vi "Puff_Release_Decay.vi"() -> (5 "Plug in titles":string[](array[string]), 7 "Plug in values":string[](array[string]))   [LabVIEW 2012]
uses:
  Globals/Meas_global.vi
  <vilib>/Analysis/baseanly.llb/Mean (DBL).vi
  <vilib>/Analysis/NI_AALBase.lvlib
  <vilib>/Analysis/NI_AALPro.lvlib
panel:
  out "Mean Concentration":dbl
  out "element":string
  out "index of element":i32
  out "Array":path[](array[path])
  out "tau":dbl(graph)
  out "tau (s)":dbl[](array[numeric])=[nan]
  in  "Median filter passes":i32=1
  in  "Median filter extent":i32=20
  in  "Normalised multiplot":bool
  in  "Cut at start":i32=200
  in  "Keep after cut":i32=2800
  in  "min threshold":dbl=4.0
  in  "Reset":bool
  out "Current Block No":i32=51
  out "Multiplot":T1(graph)
  out "XY Graph":cluster{"Time (ms)":dbl[], dbl[]}(graph)
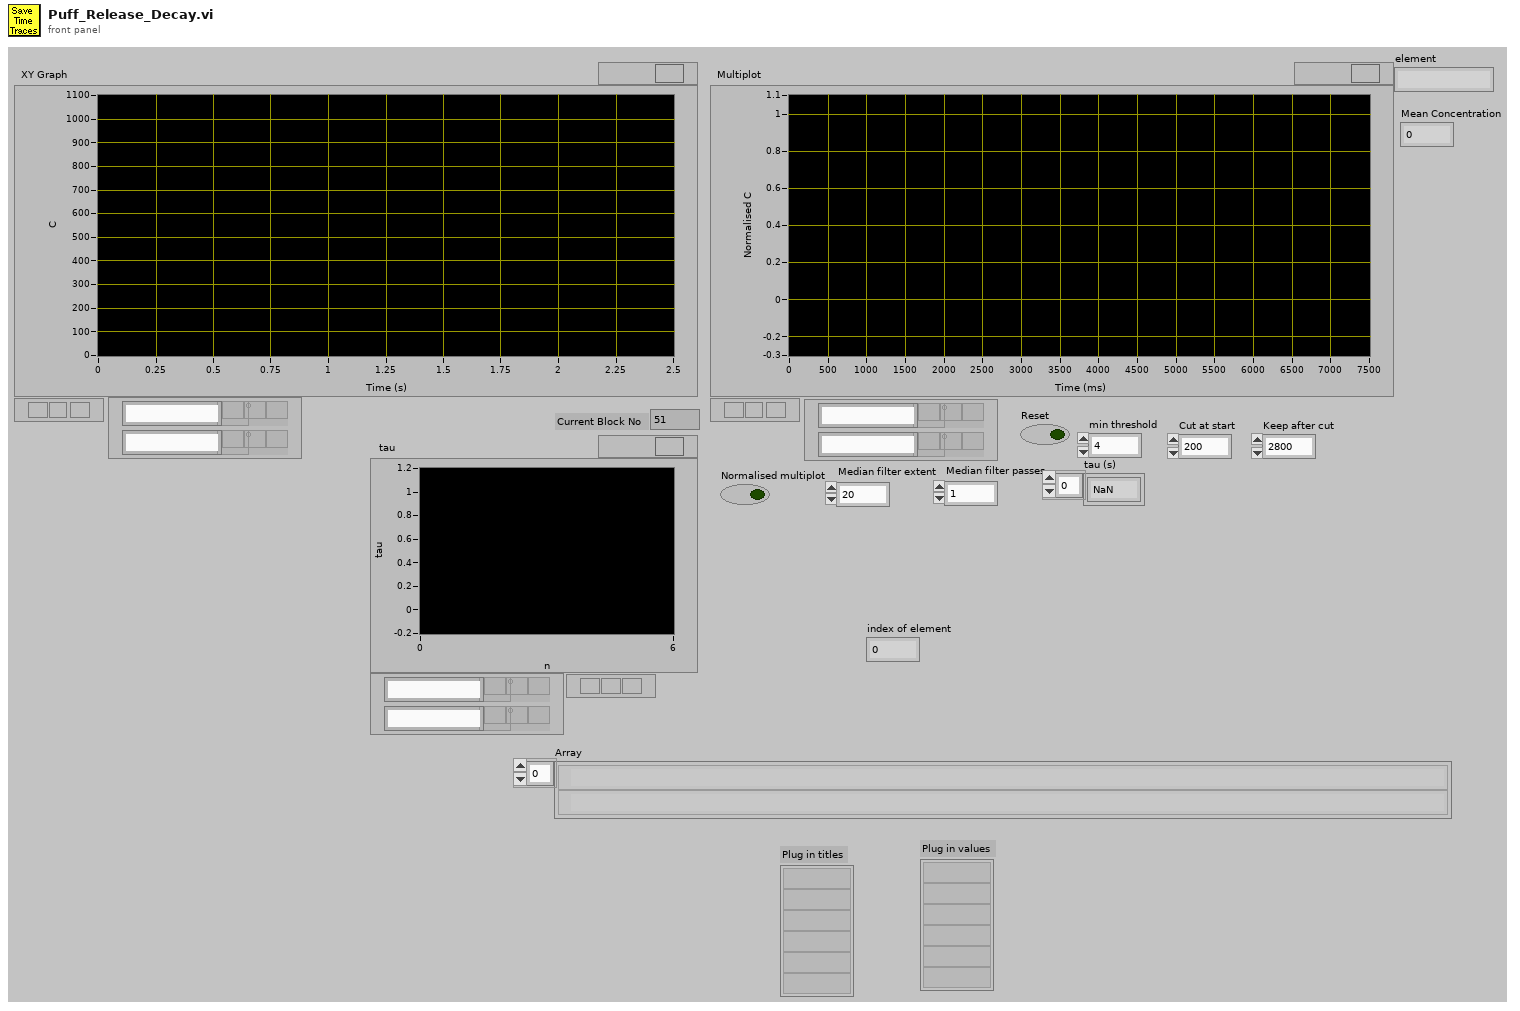
[diagram p1: front panel]
types:
  T1 = cluster{"Time (ms)":dbl[], "Y[i]=X[i]/Max|X|":dbl[]}[]
  T2 = typedef "Analysis_info_cluster.ctl" = cluster{"Colour":u32, "Inst type":T3, "Inst name":string, "Symbol":string, "Code name":string, "Extra Info":string, "Inst Array":T4, "Extra Titles":string[], "Extra Values":string[], "U":dbl, "u^2":dbl, "u^3":dbl, "u^4":dbl, "Skew_u":dbl, "Kurt_u":dbl, "Sd Error in Mean":dbl, "% u'/U":dbl, "X":dbl, "Y":dbl, "Z":dbl, "Timescale integral to 25%":dbl, "Sd Error in Variance":dbl, "Calib File":path, "Calib Constants":dbl[], "Output Position":bool, "Full Stats":bool, "Av Sampling Rate":dbl, "Av No of Samples":dbl, "Total Meas Time (s)":dbl, "ADAM Ch Name":string}
  T3 = typedef "Inst_type.ctl" = enum16{"Propeller anemometer", "Raw voltage", "Pressure Transducer", "Pitot-static tube", "Preston tube", "Hot wire", "Cross wire 1", "Cross wire 2", "Generic Linear", "Generic Polynomial", "Generic BackPoly", "Fast FID", "Thermocouple", "Cold wire", "Pulsed Wire", "LDA Vel", "LDA Tran time", "LDA Arr time"}
  T4 = typedef "Instrument_Array.ctl" = enum16{"PWA", "LDA", "Analogue"}
  T5 = typedef "Time_Trace_Cluster.ctl" = cluster{"Weighting":dbl[], "Time (s)":dbl[], "Voltage":dbl[], "Eng Values":dbl[]}
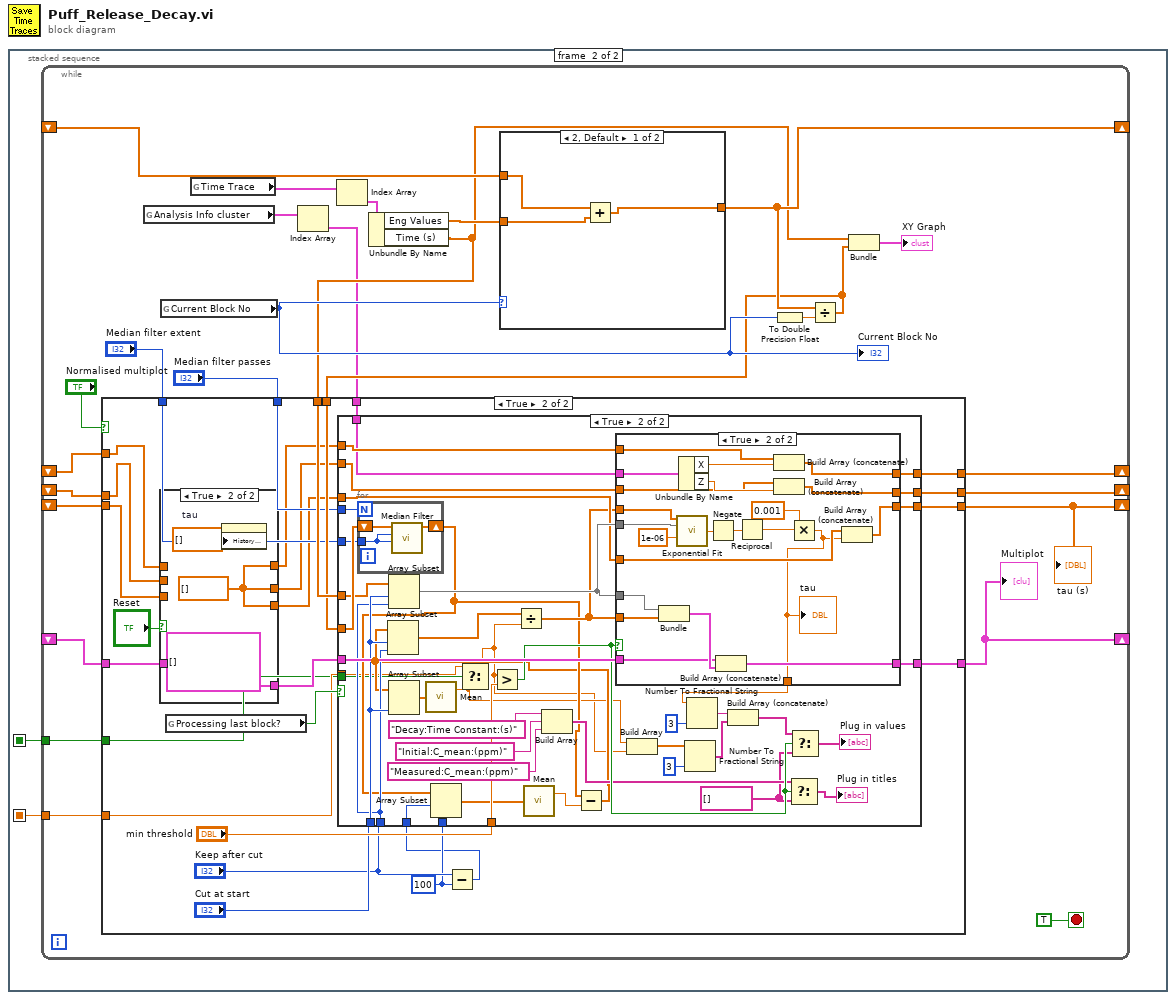
[diagram p0: block diagram]
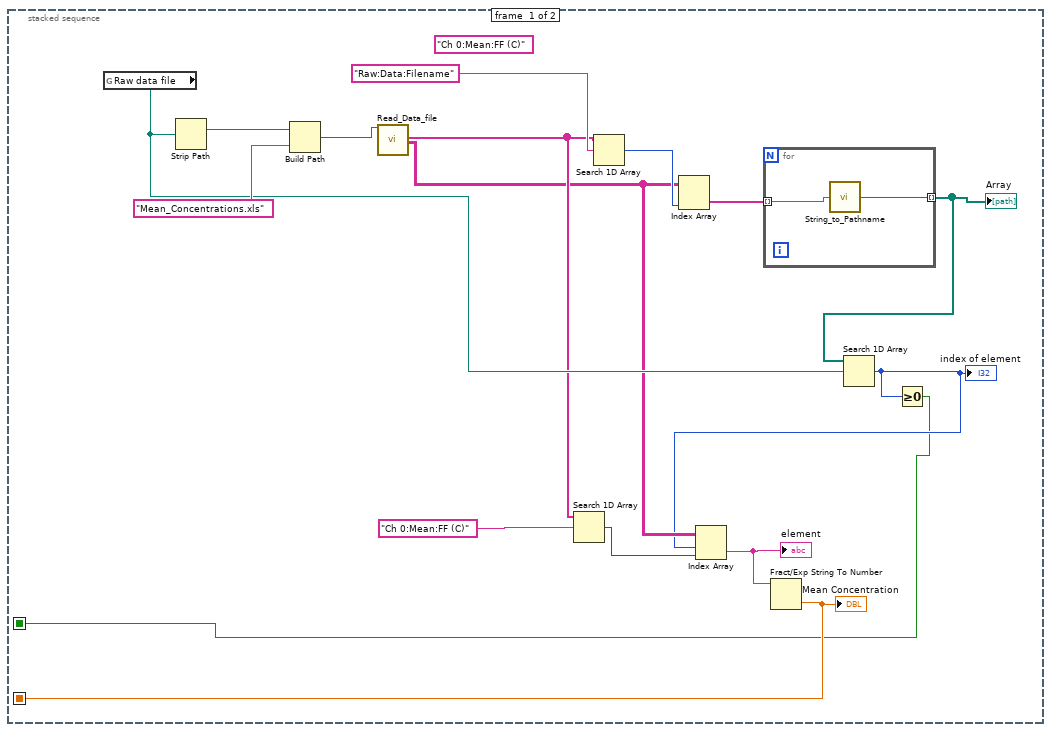
[diagram p2: hidden frame]
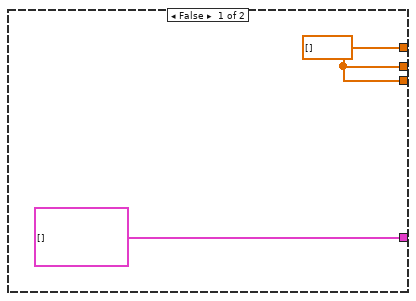
[diagram p3: hidden frame]
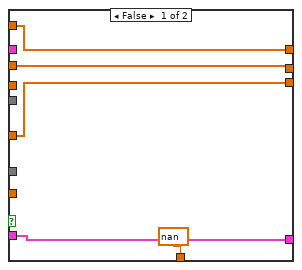
[diagram p6: hidden frame]
diagram:
  n1 = stacked-sequence {
    seq-local: [w3 _] -> [_ w20]
    seq-local: [w1 _] -> [_ w19]
    frame #0 {
      (unwired) "Ch 0:Mean:FF (C)"
      n2 = global read "Meas_global.vi" "Raw data file"() -> (w9:path)
      n3 = Strip Path(path=w9) -> (stripped path=w16:path)  [unwired: 1 out]
      n4 = Build Path(base path=w16, name or relative path="Mean_Concentrations.xls") -> (appended path=w14:path)
      n5 = call "Read_Data_file.vi"("Results file"=w14) -> ("Ch names Out"=w8:string[], "Channel Values Out"=w6:string[][])  [unwired: 9 in, 8 out]
      n6 = Search 1D Array(1D array=w8, element="Ch 0:Mean:FF (C)") -> (index of element=w5:i32)  [unwired: 1 in]
      n7 = Search 1D Array(1D array=w8, element="Raw:Data:Filename") -> (index of element=w12:i32)  [unwired: 1 in]
      n8 = Index Array(array=w6, index (col)=w12) -> (element=w11:string[])  [unwired: 1 in]
      n9 = for {
        tunnel: w11 -> [w18] mode=indexing
        tunnel: [w17] -> w10 mode=indexing
        n10 = call "String_to_Pathname.vi"("Input String"=w18) -> ("path"=w17:path)
      }
      "Array" <- w10
      n11 = Search 1D Array(1D array=w10, element=w9) -> (index of element=w2:i32)  [unwired: 1 in]
      "index of element" <- w2
      n12 = Index Array(array=w6, index (row)=w2, index (col)=w5) -> (element=w4:string)
      "element" <- w4
      n13 = Fract/Exp String To Number(string=w4) -> (number=w3:dbl)  [unwired: 3 in, 1 out]
      "Mean Concentration" <- w3
      n14 = Greater Or Equal To 0?(x=w2) -> (x >= 0?=w1:bool)
    }
    frame #1 {
      n15 = while {
        shift-right: [w39] -> _
        shift-left: _ -> [w44]
        shift-right: [w34] -> _
        shift-left: _ -> [w36]
        shift-right: [w30] -> _
        shift-left: _ -> [w27]
        shift-right: [w29] -> _
        shift-left: _ -> [w26]
        shift-right: [w28] -> _
        shift-left: _ -> [w25]
        tunnel: w20 -> [w24]
        tunnel: w19 -> [w23]
        stop <- TRUE stop-if-true
        n16 = global read "Meas_global.vi" "Analysis Info cluster"() -> (w46:T2[])
        n17 = global read "Meas_global.vi" "Current Block No"() -> (w40:i32)
        "Current Block No" <- w40
        n18 = global read "Meas_global.vi" "Time Trace"() -> (w22:T5[])
        n19 = Index Array(array=w46) -> (element=w31:T2)  [unwired: 1 in]
        n20 = Index Array(array=w22) -> (element=w21:T5)  [unwired: 1 in]
        n21 = Unbundle By Name(w21) -> ("Eng Values"=w45:dbl[], "Time (s)"=w38:dbl[])
        n22 = case shown="2, Default" w40 {
          tunnel: [w161 w164] -> w39
          tunnel: w45 -> [w163 w164]
          tunnel: w44 -> [w162 _]
          frame 2, Default {
            n23 = Add(x=w162, y=w163) -> (x+y=w161:dbl[])
          }
          frame 1 {
          }
        }
        n24 = To Double Precision Float(number=w40) -> (double precision float=w41:dbl)
        n25 = Divide(x=w39, y=w41) -> (x/y=w37:dbl[])
        n26 = case shown="True" "Normalised multiplot" {
          tunnel: w38 -> [_ w73]
          tunnel: w37 -> [_ w72]
          tunnel: w36 -> [_ w70]
          tunnel: [T1 [] w68] -> w34
          tunnel: "Median filter extent" -> [_ w65]
          tunnel: "Median filter passes" -> [_ w64]
          tunnel: w31 -> [_ w63]
          tunnel: [w47 w62] -> w30
          tunnel: [w47 w61] -> w29
          tunnel: [w47 w60] -> w28
          tunnel: w27 -> [_ w59]
          tunnel: w26 -> [_ w57]
          tunnel: w25 -> [_ w55]
          tunnel: w24 -> [_ w50]
          tunnel: w23 -> [_ w49]
          frame False {
            w47 = dbl[] []
          }
          frame True {
            w52 = 100 ("y")
            n27 = case shown="True" "Reset" {
              tunnel: [w78 T1 []] -> w69
              tunnel: w70 -> [w78 _]
              tunnel: [w77 w80] -> w58
              tunnel: [w76 w80] -> w56
              tunnel: [w75 w80] -> w54
              tunnel: w59 -> [w77 _]
              tunnel: w57 -> [w76 _]
              tunnel: w55 -> [w75 _]
              frame False {
              }
              frame True {
                w80 = dbl[] []
                n28 = property on="tau" class="WFChart (strict)"("History Data"=dbl[] []) -> ()  [unwired: 2 in, 2 out]
              }
            }
            n29 = global read "Meas_global.vi" "Processing last block?"() -> (w74:bool)
            n30 = Subtract(x="Keep after cut", y=w52) -> (x-y=w51:i32)
            n31 = case shown="True" w74 {
              tunnel: w72 -> [_ w127]
              tunnel: w73 -> [_ w115]
              tunnel: [w85 w130] -> w68
              tunnel: w69 -> [w85 w129]
              tunnel: "min threshold" -> [_ w128]
              tunnel: "Keep after cut" -> [_ w98]
              tunnel: "Cut at start" -> [_ w116]
              tunnel: w65 -> [_ w126]
              tunnel: w64 -> [_ w125]
              tunnel: w63 -> [_ w117]
              tunnel: [w84 w122] -> w62
              tunnel: [w83 w123] -> w61
              tunnel: [w82 w124] -> w60
              tunnel: w58 -> [w84 w120]
              tunnel: w56 -> [w83 w119]
              tunnel: w54 -> [w82 w118]
              tunnel: w52 -> [_ w97]
              tunnel: w51 -> [_ w96]
              tunnel: w50 -> [_ w89]
              tunnel: w49 -> [_ w88]
              frame False {
              }
              frame True {
                w99 = string[] [] ("f")
                n32 = for {
                  N: w125 -> [_]
                  shift-right: [w133] -> w94
                  shift-left: w127 -> [w132]
                  tunnel: w126 -> [w131]
                  n33 = call <vilib>:"Median Filter.vi"("right rank"=w131, "left rank"=w131, "X"=w132) -> ("Filtered X"=w133:dbl[])  [unwired: 7 in, 1 out]
                }
                n34 = Array Subset(array=w115, index=w116, length=w98) -> (w121:dbl[])
                n35 = Array Subset(array=w94, index=w96, length=w97) -> (w95:dbl[])
                n36 = call-poly <vilib>:"Mean.vi"("X"=w95) -> ("mean"=w93:dbl)  [unwired: 1 out]
                n37 = Build Array("Decay:Time Constant:(s)", "Initial:C_mean:(ppm)", "Measured:C_mean:(ppm)") -> (w103:string[])
                n38 = Subtract(x=w94, y=w93) -> (x-y=w92:dbl[])
                n39 = Array Subset(array=w92, index=w116, length=w98) -> (w113:dbl[])
                n40 = Array Subset(array=w92, length=w116) -> (w114:dbl[])  [unwired: 1 in]
                n41 = call-poly <vilib>:"Mean.vi"("X"=w114) -> ("mean"=w87:dbl)  [unwired: 1 out]
                n42 = Select(t=w89, s=w88, f=w87) -> (s? t:f=w86:dbl)
                n43 = Greater?(x=w86, y=w128) -> (0:w104:bool)
                n44 = Divide(x=w113, y=w86) -> (x/y=w112:dbl[])
                n45 = case shown="True" w104 {
                  tunnel: w121 -> [_ w160]
                  tunnel: w112 -> [_ w159]
                  tunnel: [w138 w157] -> w130
                  tunnel: w129 -> [w138 w156]
                  tunnel: [w135 w148] -> w124
                  tunnel: [w136 w147] -> w123
                  tunnel: [w137 w146] -> w122
                  tunnel: w121 -> [_ w145]
                  tunnel: w112 -> [_ w144]
                  tunnel: w117 -> [_ w143]
                  tunnel: w120 -> [w137 w142]
                  tunnel: w119 -> [w136 w141]
                  tunnel: w118 -> [w135 w140]
                  tunnel: [nan w139] -> w111
                  frame False {
                  }
                  frame True {
                    n46 = Bundle(w160, w159) -> (w158:cluster{dbl[], dbl[]})  [unwired: 1 in]
                    n47 = call <vilib>:"Exponential Fit.vi"("Y"=w144, "X"=w145, "tolerance"=1e-06) -> ("damping"=w154:dbl)  [unwired: 7 in, 5 out]
                    n48 = Unbundle By Name(w143) -> ("X"=w150:dbl, "Z"=w149:dbl)
                    n49 = Negate(x=w154) -> (-x=w153:dbl)
                    n50 = Build Array (concatenate)(w156, w158) -> (w157:T1)
                    n51 = Reciprocal(x=w153) -> (1/x=w152:dbl)
                    n52 = Build Array (concatenate)(w142, w150) -> (w146:dbl[])
                    n53 = Build Array (concatenate)(w141, w149) -> (w147:dbl[])
                    n54 = Multiply(x=0.001, y=w152) -> (x*y=w139:dbl)
                    "tau" <- w139
                    n55 = Build Array (concatenate)(w140, w139) -> (w148:dbl[])
                  }
                }
                n56 = Build Array(w87, w86) -> (w90:dbl[])
                n57 = Number To Fractional String(number=w90, precision (6)=i16 3) -> (F-format string=w105:string[])  [unwired: 2 in]
                n58 = Number To Fractional String(number=w111, precision (6)=i16 3) -> (F-format string=w110:string)  [unwired: 2 in]
                n59 = Build Array (concatenate)(w110, w105) -> (w100:string[])
                n60 = Select(t=w103, s=w104, f=w99) -> (s? t:f=→"Plug in titles":string[])
                n61 = Select(t=w100, s=w104, f=w99) -> (s? t:f=→"Plug in values":string[])
              }
            }
          }
        }
        "Multiplot" <- w34
        "tau (s)" <- w28
        n62 = Bundle("Time (s)"=w38, w37) -> (→"XY Graph":cluster{"Time (s)":dbl[], dbl[]})  [unwired: 1 in]
      }
    }
  }
